vi "Get MouseEventArgs.vi"(8 "error in (no error)":errorcluster, 11 "MouseEventArgs in":refnum<class "MouseEventArgs.lvclass">) -> (0 "error out":errorcluster, 2 "MouseEventArgs":refnum<k24>, 3 "MouseEventArgs out":refnum<class "MouseEventArgs.lvclass">)   [LabVIEW 2023, in "SourceGrid.lvlib" / "MouseEventArgs.lvclass"]
uses:
  MouseEventArgs.lvclass
  System.Windows.Forms
  MouseEventArgs.lvclass/MouseEventArgs.ctl
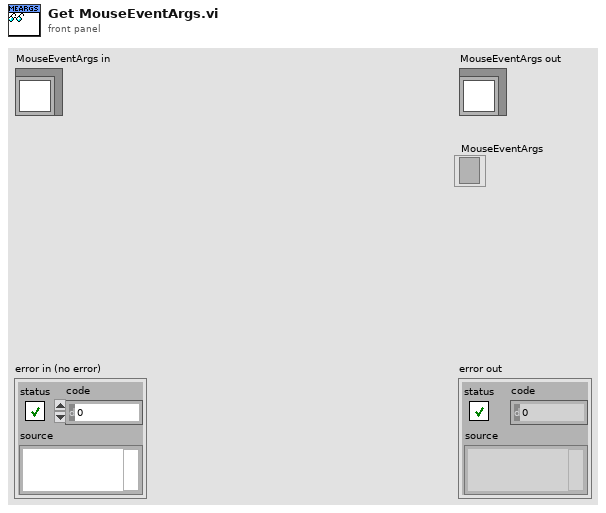
[diagram p1: front panel]
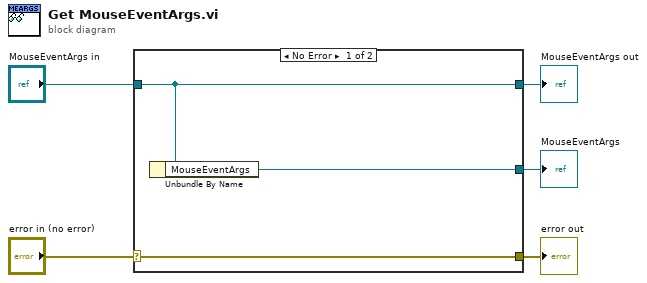
[diagram p0: block diagram]
diagram:
  n1 = case shown="No Error" "error in (no error)" {
    selector: "error in (no error)" -> [w8 w9]
    tunnel: [w8 w9] -> w4
    tunnel: [w7 w10] -> w2
    tunnel: "MouseEventArgs in" -> [w7 w10]
    tunnel: [w6 _] -> w1
    frame No Error {
      n2 = Unbundle By Name(w7) -> ("MouseEventArgs"=w6:refnum<k24>)
    }
    frame Error {
    }
  }
  "error out" <- w4
  "MouseEventArgs out" <- w2
  "MouseEventArgs" <- w1
